vi "Get Maximum Data Length.vi"(11 "variant in":variant) -> (1 "maximum data length":i32, 3 "variant out":variant)   [LabVIEW 2017]
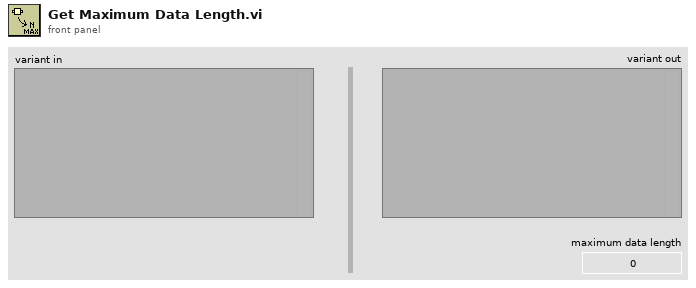
[diagram p1: front panel]
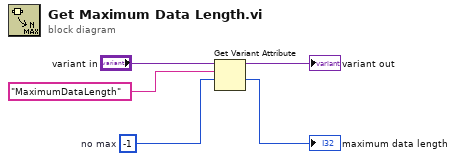
[diagram p0: block diagram]
diagram:
  w4 = -1  # no max
  n1 = Get Variant Attribute(Variant="variant in", name="MaximumDataLength", default value (empty Variant)=w4) -> (duplicate Variant=→"variant out":variant, value=→"maximum data length":i32)  [unwired: 1 in, 2 out]
